vi "Change Tunnel Modes to Fix Wires.vi"(8 "error in (no error)":errorcluster, 10 "All Tunnels (before wiring)":refnum<vi>[](array[refnum]), 11 "VI":refnum<vi>) -> (0 "error out":errorcluster, 3 "dup VI":refnum<vi>)   [LabVIEW 2016]
uses:
  <vilib>/Utility/traverseref.llb/TRef TravTarget.ctl
  <vilib>/Utility/traverseref.llb/VI Scripting - Traverse.lvlib
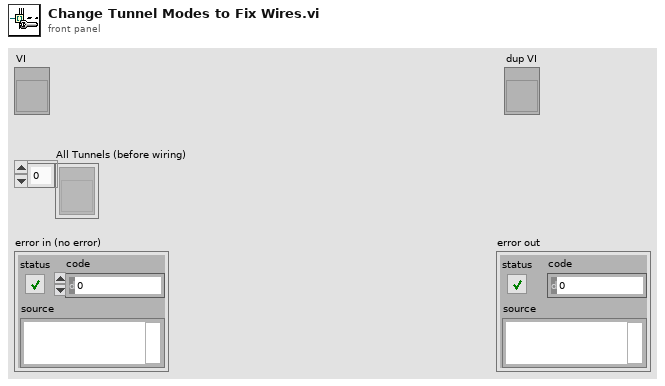
[diagram p1: front panel]
types:
  T1 = typedef "TRef TravTarget.ctl" = enum16{"FP", "BD", "Other"}
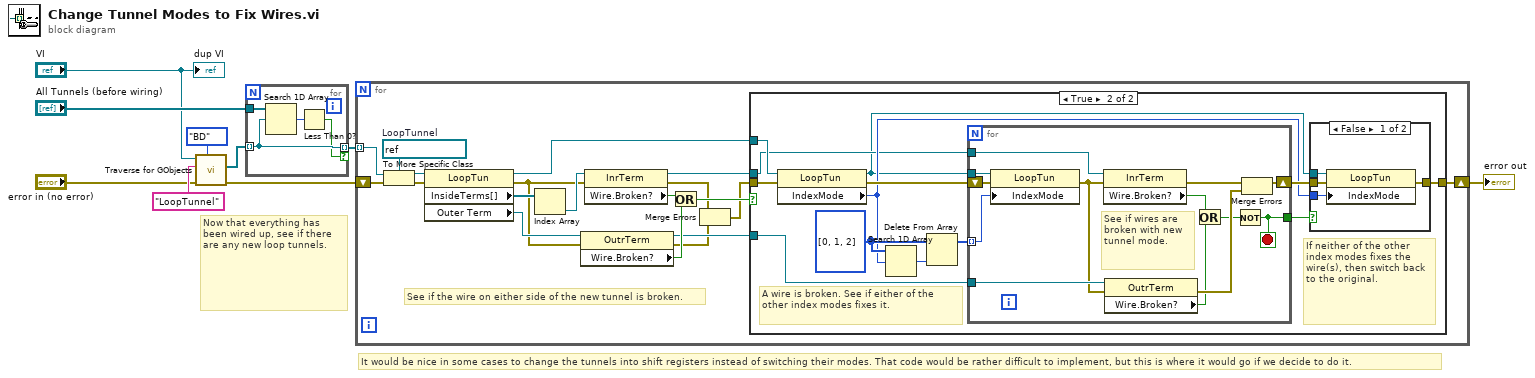
[diagram p0: block diagram]
diagram:
  # "It would be nice in some cases to change the tunnels into shift registers instead of switching their modes. That code would be rather difficult to implement, but this is where it would go if we decide to do it."
  # "Now that everything has been wired up, see if there are any new loop tunnels."
  n1 = call <vilib>:"Traverse for GObjects.vi"("Traverse Target"=TRef_TravTarget."BD", "error in (no error)"="error in (no error)", "Class Name"="LoopTunnel", "VI Refnum"="VI") -> ("error out"=w7:errorcluster, "References"=w6:refnum<vi>[])  [unwired: 4 in, 2 out]
  n2 = for {
    tunnel: w6 -> [w11] mode=indexing
    tunnel: "All Tunnels (before wiring)" -> [w13]
    tunnel: [w11] -> w8 mode=indexing if=w10
    n3 = Search 1D Array(1D array=w13, element=w11) -> (index of element=w12:i32)  [unwired: 1 in]
    n4 = Less Than 0?(x=w12) -> (x < 0?=w10:bool)
  }
  n5 = for {
    shift-right: [w32] -> w3
    shift-left: w7 -> [w30]
    tunnel: w8 -> [w31] mode=indexing
    w29 = refnum<vi> refnum  # LoopTunnel
    # "See if the wire on either side of the new tunnel is broken."
    n6 = To More Specific Class(target class=w29, reference=w31, error in=w30) -> (specific class reference=w28:refnum<vi>, error out=w27:errorcluster)
    n7 = property class="LoopTun"(reference=w28, error in=w27) -> (reference out=w19:refnum<vi>, error out=w23:errorcluster, "InsideTerms[]"=w26:refnum<vi>[], "Outer Term"=w24:refnum<vi>)
    n8 = Index Array(array=w26) -> (element=w25:refnum<vi>)  [unwired: 1 in]
    n9 = property class="OutrTerm"(reference=w24, error in=w23) -> (reference out=w17:refnum<vi>, error out=w16:errorcluster, "Wire.Broken?"=w21:bool)
    n10 = property class="InrTerm"(reference=w25, error in=w23) -> (reference out=w18:refnum<vi>, error out=w15:errorcluster, "Wire.Broken?"=w22:bool)
    n11 = Or(x=w22, y=w21) -> (x .or. y?=w20:bool)
    n12 = Merge Errors(w15, w16) -> (w14:errorcluster)
    n13 = case shown="True" w20 {
      tunnel: w14 -> [w33 w46]
      tunnel: [w33 w45] -> w32
      tunnel: w19 -> [_ w37]
      tunnel: w18 -> [_ w36]
      tunnel: w17 -> [_ w34]
      frame False {
        # "Wire is not broken...leave it alone."
      }
      frame True {
        w43 = i32[] [0, 1, 2]
        # "If neither of the other index modes fixes the wire(s), then switch back to the original."
        # "A wire is broken. See if either of the other index modes fixes it."
        n14 = property class="LoopTun"(reference=w37, error in=w46) -> (reference out=w35:refnum<vi>, error out=w42:errorcluster, "IndexMode"=w38:u32)
        n15 = Search 1D Array(1D array=w43, element=w38) -> (index of element=w44:i32)  [unwired: 1 in]
        n16 = Delete From Array(array=w43, index=w44) -> (array with subset deleted=w41:i32[])  [unwired: 1 in, 1 out]
        n17 = for {
          shift-right: [w56] -> w39
          shift-left: w42 -> [w64]
          tunnel: w41 -> [w63] mode=indexing
          tunnel: w36 -> [w62]
          tunnel: [w60] -> w40
          tunnel: w35 -> [w59]
          tunnel: w34 -> [w58]
          stop <- w60 stop-if-true
          # "See if wires are broken with new tunnel mode."
          n18 = property class="LoopTun"(reference=w59, error in=w64, "IndexMode"=w63) -> (error out=w57:errorcluster)  [unwired: 1 out]
          n19 = property class="InrTerm"(reference=w62, error in=w57) -> (error out=w61:errorcluster, "Wire.Broken?"=w54:bool)  [unwired: 1 out]
          n20 = property class="OutrTerm"(reference=w58, error in=w57) -> (error out=w55:errorcluster, "Wire.Broken?"=w53:bool)  [unwired: 1 out]
          n21 = Or(x=w54, y=w53) -> (x .or. y?=w52:bool)
          n22 = Not(x=w52) -> (.not. x?=w60:bool)
          n23 = Merge Errors(w61, w55) -> (w56:errorcluster)
        }
        n24 = case shown="False" w40 {
          tunnel: w39 -> [w50 w51]
          tunnel: [w49 w51] -> w45
          tunnel: w35 -> [w48 _]
          tunnel: w38 -> [w47 _]
          frame False {
            n25 = property class="LoopTun"(reference=w48, error in=w50, "IndexMode"=w47) -> (error out=w49:errorcluster)  [unwired: 1 out]
          }
          frame True {
          }
        }
      }
    }
  }
  "error out" <- w3
  "dup VI" <- "VI"
